vi "Mode Test Shutdown.vi"(7 "Sequence Context In":refnum<k7>, 8 "error in":errorcluster, 9 "Test Mode":u16, 10 "LV PPS Config":T1={"VISA Resource"="", "Voltage Level (0.0 V)"=12.0, "CURRent Limit (0.0 A)"=6.0, "OVP LEVEL (0V)"=15.0, "Enable OVP (T: Enable)"=FALSE, "OCP LEVEL (0A)"=8.0, "Enable OCP (T: Enable)"=TRUE, "Value Out"="", "Value In"="", "Actual Voltage Level (V)"=-0.11, "Actual Current Limit (A)"=0.0, "Select Instrument"="", "Enable Output"=TRUE, "PPS Operation"=enum."Configure", "Type"=0} {"Type" items=["Voltage", "Current"]; "Actual Current Limit (A)" format="%.2f"; "Actual Voltage Level (V)" format="%.2f"; "OCP LEVEL (0A)" format="%.2f"; "OVP LEVEL (0V)" format="%.2f"; "Voltage Level (0.0 V)" format="%.2f"}, 11 "HV PPS Config":T1={"VISA Resource"="", "Voltage Level (0.0 V)"=48.0, "CURRent Limit (0.0 A)"=150.0, "OVP LEVEL (0V)"=55.0, "Enable OVP (T: Enable)"=FALSE, "OCP LEVEL (0A)"=160.0, "Enable OCP (T: Enable)"=TRUE, "Value Out"="", "Value In"="", "Actual Voltage Level (V)"=-0.11, "Actual Current Limit (A)"=0.0, "Select Instrument"="", "Enable Output"=TRUE, "PPS Operation"=enum."Configure", "Type"=0} {"Type" items=["Voltage", "Current"]; "Actual Current Limit (A)" format="%.2f"; "Actual Voltage Level (V)" format="%.2f"; "OCP LEVEL (0A)" format="%.2f"; "OVP LEVEL (0V)" format="%.2f"; "Voltage Level (0.0 V)" format="%.2f"}) -> (0 "error out":errorcluster)   [LabVIEW 2023, in "HardwareAbstractionLayer_LVOOP.lvlib" / "Wait Monitor.lvclass"]
uses:
  Wait Monitor.lvclass
  PowerSupply/Teststand/Control/PPS StepType Control.ctl
  Teststand Steptypes/CAN/STP/Steptypes/Control/STP Data.ctl
  CAN/CAN Application Protocols/STP Protocol_class/Ctrls/STP CMD.ctl
  Teststand Steptypes/DAQ/Relay Output/Control/Relay Output.ctl
  Teststand/Teststand.lvclass
  CAN/CAN Application Protocols/STP Protocol_class/STP Protocol.lvclass
  Teststand Steptypes/LTT_TeststandSteptypes.lvlib
  PowerSupply/PowerSupply.lvclass
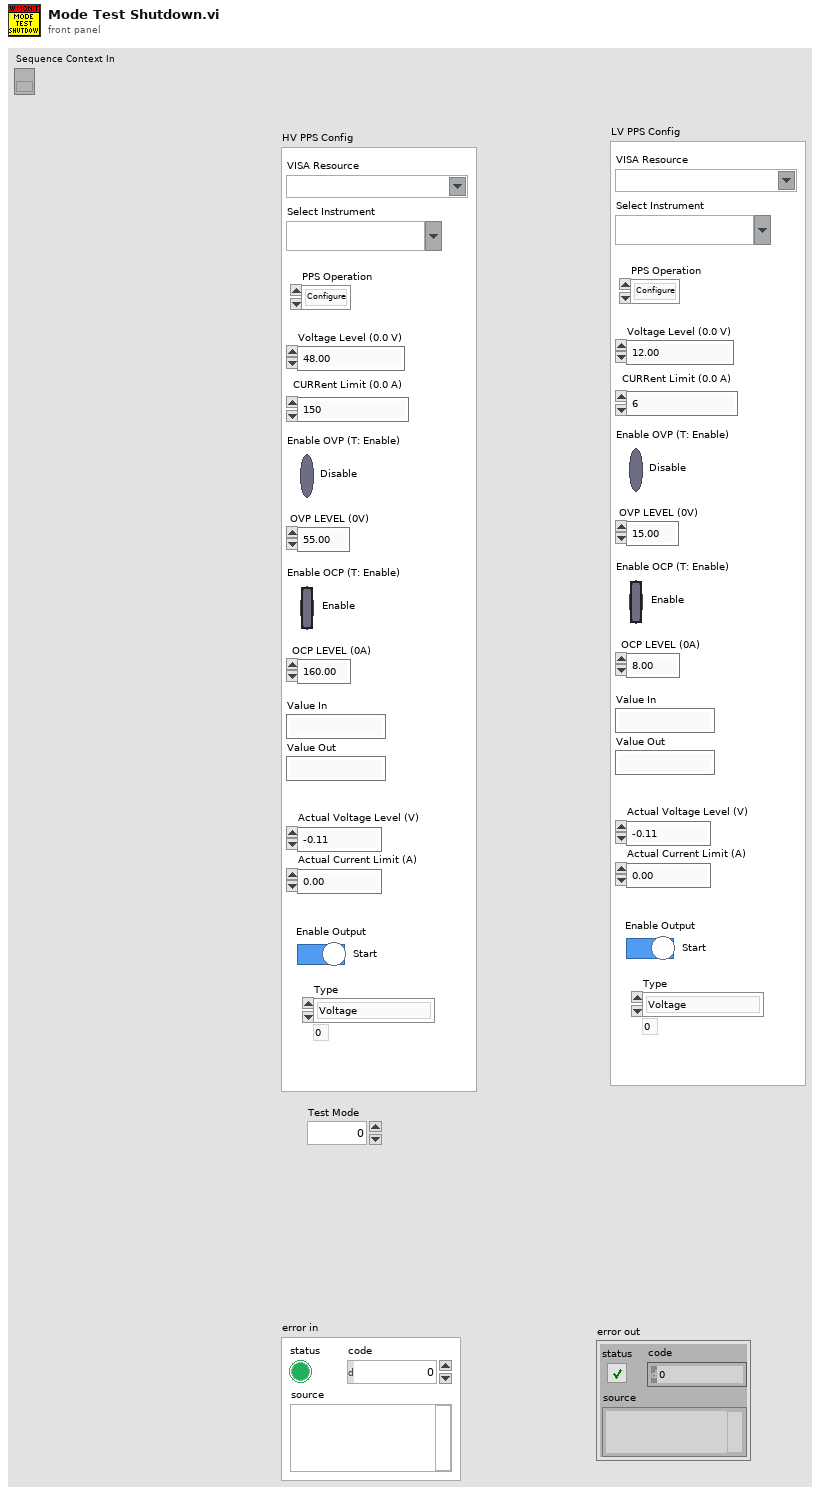
[diagram p1: front panel]
types:
  T1 = typedef "HardwareAbstractionLayer_LVOOP.lvlib/PowerSupply.lvclass/PPS StepType Control.ctl" = cluster{"VISA Resource":refnum<visa-resource-name>, "Voltage Level (0.0 V)":dbl, "CURRent Limit (0.0 A)":dbl, "OVP LEVEL (0V)":dbl, "Enable OVP (T: Enable)":bool, "OCP LEVEL (0A)":dbl, "Enable OCP (T: Enable)":bool, "Value Out":string, "Value In":string, "Actual Voltage Level (V)":dbl, "Actual Current Limit (A)":dbl, "Select Instrument":string, "Enable Output":bool, "PPS Operation":enum32{"Init", "Self Test", "Configure", "Measure", "Close"}, "Type":u16}
  T2 = typedef "HardwareAbstractionLayer_LVOOP.lvlib/CAN Application Protocols Lib.lvlib/STP Protocol.lvclass/STP CMD.ctl" = u8
  T3 = typedef "LTT_TeststandSteptypes.lvlib/STP Data.ctl" = cluster{"ECU CAN Port":string, "CMD":T2, "CAN Write Data":u8[], "Response Decoder":enum16{"String", "Number", "Boolean"}, "String":cluster{"Start Index":i32, "Length":i32}, "Number":cluster{"MSB Index":i32, "LSB Index":i32}, "Boolean":cluster{"Index":i32, "Bool":cluster{"7":bool, "6":bool, "5":bool, "4":bool, "3":bool, "2":bool, "1":bool, "0":bool, "7 Enabled":bool, "6 Enabled":bool, "5 Enabled":bool, "4 Enabled":bool, "3 Enabled":bool, "2 Enabled":bool, "1 Enabled":bool, "0 Enabled":bool}}}
  T4 = enum32{"Init", "Self Test", "Configure", "Measure", "Close"}
  T5 = typedef "LTT_TeststandSteptypes.lvlib/Relay Output.ctl" = cluster{"Signal Name List":cluster{"Signal Name":string, "Enable Output":bool}[]}
  T6 = typedef "HardwareAbstractionLayer_LVOOP.lvlib/Teststand.lvclass/Teststand Status Control.ctl" = cluster{"Terminating or Aborting":bool, "Stop":bool, "Socket Count":i16, "Selected Sockets":i16[]}
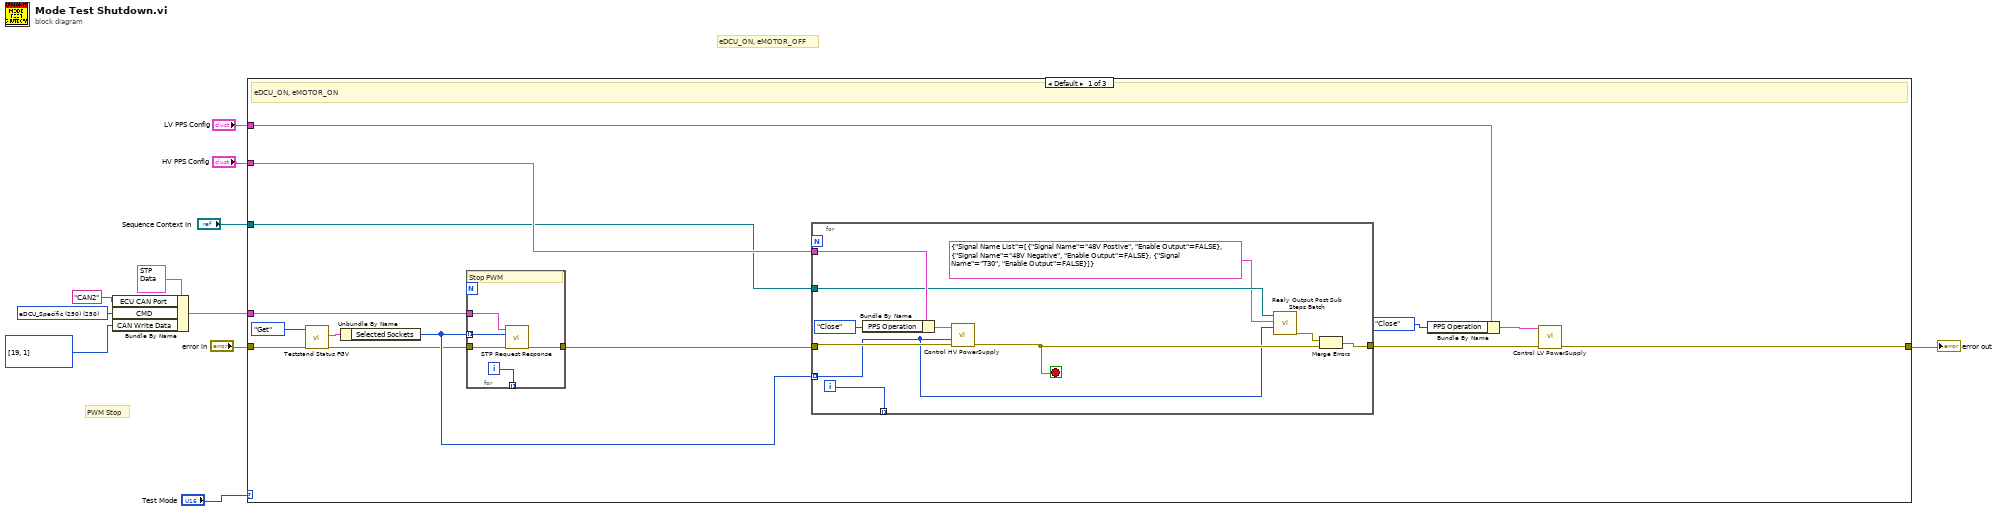
[diagram p0: block diagram]
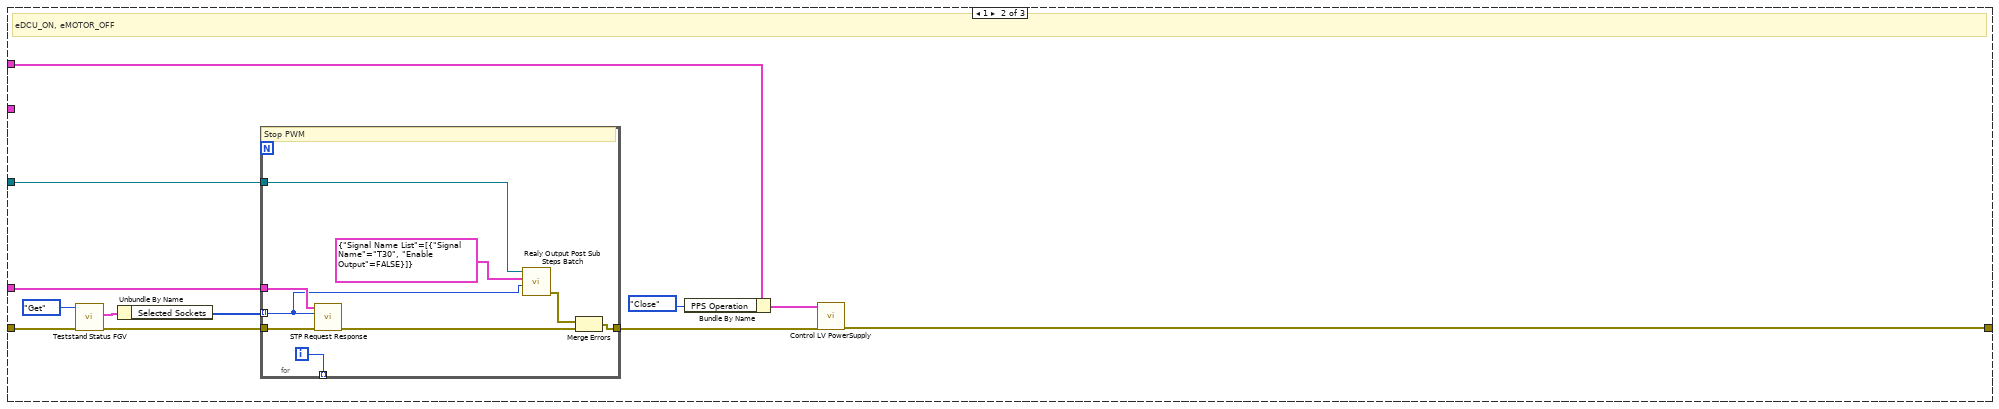
[diagram p2: hidden frame]
diagram:
  w5 = T2 250 items=["TSW_VERSION(130)"=130, "WAIT_EVENT(132)"=132, "SEQUENCER(133)"=133, "TSW_RESET(150)"=150, "CONFIG_ECU(151)"=151, "TEST_CORE (152)"=152, "TEST_WATCHDOG (153)"=153, "TEST_MONITORING (154)"=154, "READ_MEMORY (162)"=162, "WRITE_ERASE_MEMORY (164)"=164, "COMM_EXTERNAL (190)"=190, "COMM_INTERNAL (195)"=195, "GET_ANALOG_INPUT (210)"=210, "GET_DIGITAL_INPUT (211)"=211, "GET_FREQUENCY_INPUT (212)"=212, "TEST_INPUT_STRUCTURE (214)"=214, "GENERATE_OUTPUT_SIGNAL (220)"=220, "GENERATE_SYNCHRONIZED_OUTPUT_SIGNALS (221)"=221, "eDCU_Specific (250)"=250] ("CMD")
  # "PWM Stop"
  # "eDCU_ON, eMOTOR_OFF"
  n1 = Bundle By Name(cluster=T3 {"ECU CAN Port"="CAN2", "CMD"=130, "CAN Write Data"=[], "Response Decoder"=enum."String", "String"={"Start Index"=0, "Length"=-1}, "Number"={"MSB Index"=0, "LSB Index"=1}, "Boolean"={"Index"=0, "Bool"={"7"=FALSE, "6"=FALSE, "5"=FALSE, "4"=FALSE, "3"=FALSE, "2"=FALSE, "1"=FALSE, "0"=FALSE, "7 Enabled"=FALSE, "6 Enabled"=FALSE, "5 Enabled"=FALSE, "4 Enabled"=FALSE, "3 Enabled"=FALSE, "2 Enabled"=FALSE, "1 Enabled"=FALSE, "0 Enabled"=FALSE}}} ("STP Data in"), "ECU CAN Port"="CAN2", "CMD"=w5, "CAN Write Data"=u8[] [19, 1]) -> (w3:T3)
  n2 = case shown="Default" "Test Mode" {
    tunnel: "error in" -> [w23 w51 w63]
    tunnel: [w14 w43 w63] -> w2
    tunnel: "HV PPS Config" -> [w22 _ _]
    tunnel: "LV PPS Config" -> [w21 w50 _]
    tunnel: w3 -> [w17 w45 _]
    tunnel: "Sequence Context In" -> [w13 w42 _]
    frame Default {
      # "eDCU_ON, eMOTOR_ON"
      n3 = call "Teststand Status FGV.vi"("error in"=w23, "Option"=enum16{"Set", "Get"}."Get") -> ("error out"=w19:errorcluster, "Teststand Status Out"=w24:T6)  [unwired: 8 in]
      n4 = Unbundle By Name(w24) -> ("Selected Sockets"=w20:i16[])
      n5 = for {
        tunnel: [w29] -> _ mode=indexing
        tunnel: w20 -> [w28] mode=indexing
        tunnel: [w30] -> w18
        tunnel: w19 -> [w27]
        tunnel: w17 -> [w26]
        i -> [w29]
        # "Stop PWM"
        n6 = call "STP Request Response.vi"("error in"=w27, "Socket No"=w28, "STP Data in"=w26) -> ("error out"=w30:errorcluster)  [unwired: 5 in, 3 out]
      }
      n7 = for {
        tunnel: [w35] -> w16
        tunnel: w20 -> [w33] mode=indexing
        tunnel: w22 -> [w41]
        tunnel: [w38] -> _ mode=indexing
        tunnel: w18 -> [w37]
        tunnel: w13 -> [w32]
        i -> [w38]
        stop <- w36 stop-if-true
        n8 = Bundle By Name(cluster=w41, "PPS Operation"=T4."Close") -> (w40:T1)
        n9 = call "Control HV PowerSupply.vi"("error in"=w37, "Socket Index"=w33, "PPS Config In"=w40) -> ("error out"=w36:errorcluster)  [unwired: 6 in, 2 out]
        n10 = call "Realy Output Post Sub Steps Batch.vi"("Socket No"=w33, "RelayOutputWrite"=T5 {"Signal Name List"=[{"Signal Name"="48V Postive", "Enable Output"=FALSE}, {"Signal Name"="48V Negative", "Enable Output"=FALSE}, {"Signal Name"="T30", "Enable Output"=FALSE}]}, "Sequence Context In"=w32) -> ("error out"=w34:errorcluster)  [unwired: 6 in, 2 out]
        n11 = Merge Errors(w34, w36) -> (w35:errorcluster)
      }
      n12 = Bundle By Name(cluster=w21, "PPS Operation"=T4."Close") -> (w15:T1)
      n13 = call "Control LV PowerSupply.vi"("error in"=w16, "PPS Config In"=w15) -> ("error out"=w14:errorcluster)  [unwired: 7 in, 2 out]
    }
    frame 1 {
      # "eDCU_ON, eMOTOR_OFF"
      n14 = call "Teststand Status FGV.vi"("error in"=w51, "Option"=enum16{"Set", "Get"}."Get") -> ("error out"=w47:errorcluster, "Teststand Status Out"=w52:T6)  [unwired: 8 in]
      n15 = Unbundle By Name(w52) -> ("Selected Sockets"=w48:i16[])
      n16 = for {
        tunnel: [w61] -> _ mode=indexing
        tunnel: w48 -> [w56] mode=indexing
        tunnel: [w55] -> w46
        tunnel: w47 -> [w60]
        tunnel: w45 -> [w59]
        tunnel: w42 -> [w57]
        i -> [w61]
        # "Stop PWM"
        n17 = call "STP Request Response.vi"("error in"=w60, "Socket No"=w56, "STP Data in"=w59) -> ("error out"=w62:errorcluster)  [unwired: 5 in, 3 out]
        n18 = call "Realy Output Post Sub Steps Batch.vi"("Socket No"=w56, "RelayOutputWrite"=T5 {"Signal Name List"=[{"Signal Name"="T30", "Enable Output"=FALSE}]}, "Sequence Context In"=w57) -> ("error out"=w54:errorcluster)  [unwired: 6 in, 2 out]
        n19 = Merge Errors(w54, w62) -> (w55:errorcluster)
      }
      n20 = Bundle By Name(cluster=w50, "PPS Operation"=T4."Close") -> (w44:T1)
      n21 = call "Control LV PowerSupply.vi"("error in"=w46, "PPS Config In"=w44) -> ("error out"=w43:errorcluster)  [unwired: 7 in, 2 out]
    }
    frame 0 {
      # "eDCU_OFF, eMOTOR_OFF"
    }
  }
  "error out" <- w2
